vi "ingest.tabular_set_timestamp_epoch.vi"(8 "error in":errorcluster, 11 "TabularIngestStaging in":refnum<class "TabularIngestStaging.lvclass">) -> (0 "error out":errorcluster, 3 "TabularIngestStaging out":refnum<class "TabularIngestStaging.lvclass">)   [LabVIEW 2020, in "TabularIngestStaging.lvclass"]
doc: "Specifies that row timestamps are numeric epoch values in the named column, in a given time unit."
uses:
  TabularIngestStaging.lvclass
  TabularIngestStaging.lvclass/TabularIngestStaging.ctl
  client.lvlib
panel:
  in  "column":string
  in  "time_unit":i32
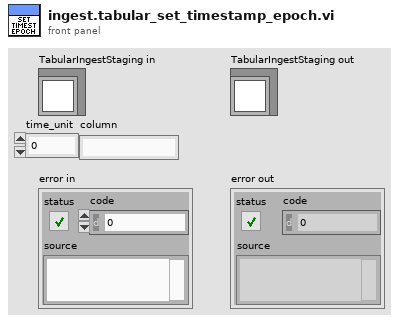
[diagram p1: front panel]
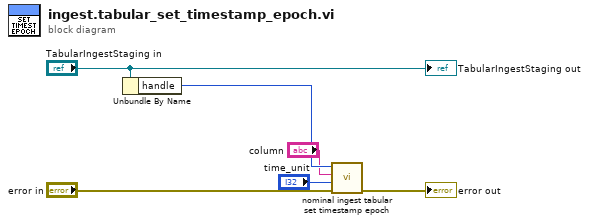
[diagram p0: block diagram]
diagram:
  n1 = Unbundle By Name("TabularIngestStaging in") -> ("handle"=w4:i32)
  n2 = call "nominal ingest tabular set timestamp epoch.vi"("error in (no error)"="error in", "time_unit"="time_unit", "column"="column", "staging"=w4) -> ("error out"=→"error out":errorcluster)  [unwired: 6 in, 1 out]
  "TabularIngestStaging out" <- "TabularIngestStaging in"
